vi "StartTrial.vi"(8 "error in (no error)":errorcluster, 11 "TrialBasedExperiment in":refnum<class "MultDimExperiment.lvclass">) -> (0 "error out":errorcluster, 3 "TrialBasedExperiment out":refnum<class "MultDimExperiment.lvclass">)   [LabVIEW 2011, in "MultDimExperiment.lvclass"]
uses:
  MultDimExperiment.lvclass
  Trial Based Experiment Statechart/PassiveExperiment/PassiveExperiment.lvclass
  Matlab API/Matlab API.lvlib
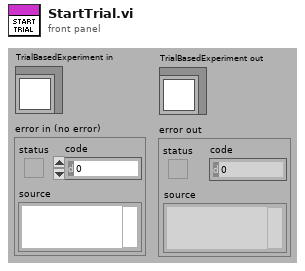
[diagram p1: front panel]
types:
  T1 = cluster{"Intertrial":dbl, "AcquireFixation":dbl, "HoldFixation":dbl, "DelayPeriod":dbl, "ResponsePeriod":dbl}
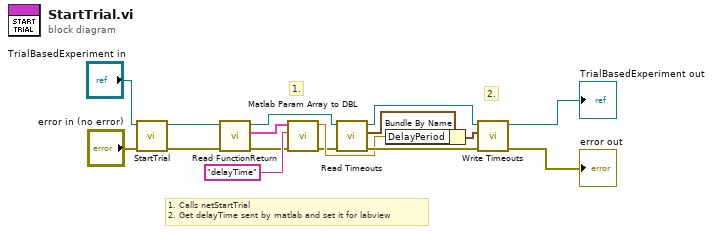
[diagram p0: block diagram]
diagram:
  # "1. Calls netStartTrial\n2. Get delayTime sent by matlab and set it for labview"
  # "2."
  # "1."
  n1 = call-parent "StartTrial.vi"("error in (no error)"="error in (no error)", "TrialBasedExperiment in"="TrialBasedExperiment in") -> ("error out"=w3:errorcluster, "TrialBasedExperiment out"=w4:refnum<class "MultDimExperiment.lvclass">)  [unwired: 8 in]
  n2 = call-dynamic "Read FunctionReturn.vi"("error in (no error)"=w3, "MatlabExperiment in"=w4) -> ("error out"=w6:errorcluster, "FunctionReturn"=w11:cluster{"Name":string, "Data":variant}[], "MatlabExperiment out"=w14:refnum<class "MultDimExperiment.lvclass">)  [unwired: 7 in]
  n3 = call "Matlab Param Array to DBL.vi"("error in (no error)"=w6, "Name"="delayTime", "Matlab Param Array"=w11) -> ("error out"=w5:errorcluster, "data"=w8:dbl)  [unwired: 7 in]
  n4 = call-dynamic "Read Timeouts.vi"("error in (no error)"=w5, "TrialBasedExperiment in"=w14) -> ("error out"=w12:errorcluster, "Timeouts"=w9:T1, "TrialBasedExperiment out"=w13:refnum<class "MultDimExperiment.lvclass">)  [unwired: 7 in]
  n5 = Bundle By Name(cluster=w9, "DelayPeriod"=w8) -> (w7:T1)
  n6 = call-dynamic "Write Timeouts.vi"("error in (no error)"=w12, "Timeouts"=w7, "TrialBasedExperiment in"=w13) -> ("error out"=→"error out":errorcluster, "TrialBasedExperiment out"=→"TrialBasedExperiment out":refnum<class "MultDimExperiment.lvclass">)  [unwired: 7 in]
